vi "CLD 1 Elapsed Time Express Front Panel.vi"() -> ()   [LabVIEW 2009]
doc: "LabVIEW CLD 1 Exercise"
panel:
  out "error out":errorcluster
  in  "error in":errorcluster
  out "Elapsed Time":string
  out "Time has Elapsed":bool
  in  "Auto Reset":bool
  in  "Reset Button":bool
  in  "Stop VI":bool
  in  "Time Target (s)":dbl
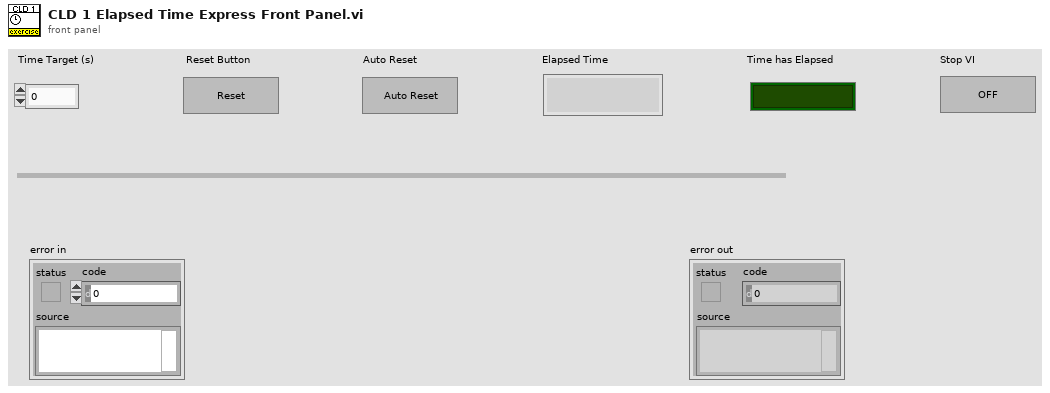
[diagram p1: front panel]
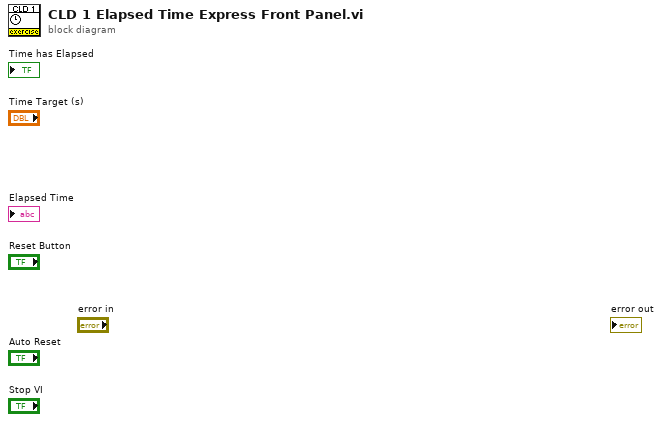
[diagram p0: block diagram]
diagram:
